vi "FTW-File-TextWrite.vi"(0 "Filepath":path, 5 "Text to Write":string, 7 "Mode":enum16{"Overwrite", "Append"}(ring), 11 "error in":errorcluster) -> (4 "Filepath out":path, 15 "error out":errorcluster)   [LabVIEW 2015]
panel:
  # "Inputs"
  # "Outputs"
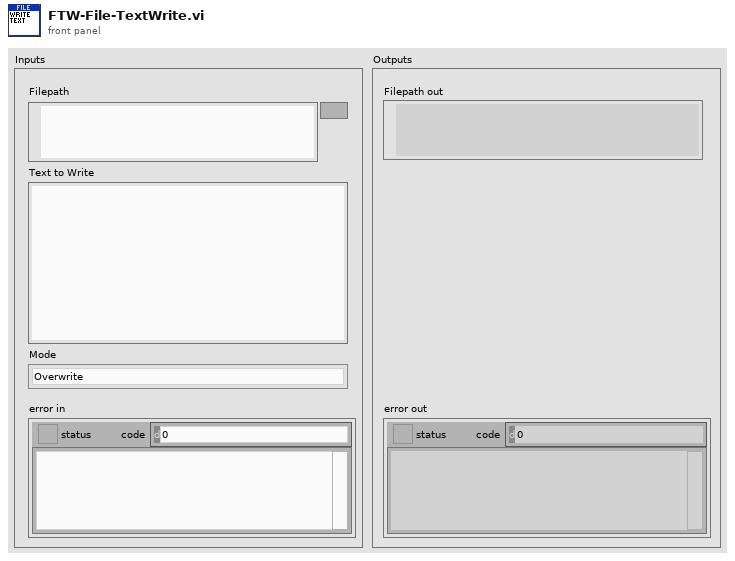
[diagram p1: front panel]
types:
  T1 = enum16{"open", "replace", "create", "open or create", "replace or create", "replace or create with confirmation"}
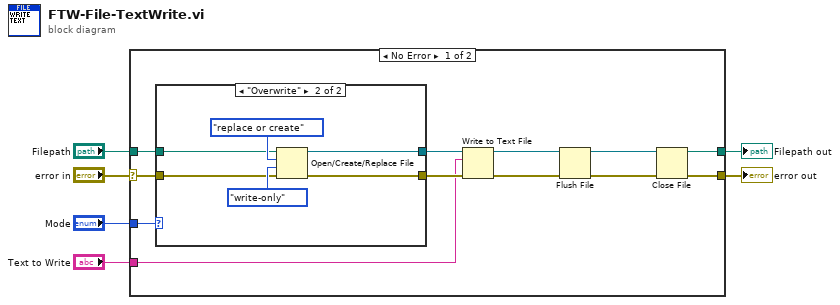
[diagram p0: block diagram]
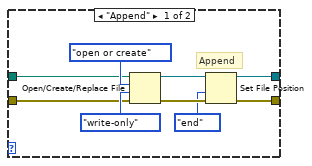
[diagram p2: hidden frame]
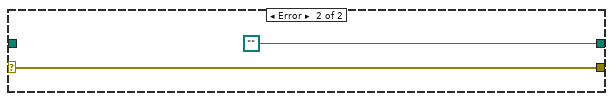
[diagram p3: hidden frame]
diagram:
  n1 = case shown="No Error" "error in" {
    selector: "error in" -> [w10 w34]
    tunnel: "Text to Write" -> [w15 _]
    tunnel: "Filepath" -> [w14 _]
    tunnel: [w13 path ""] -> w4
    tunnel: [w12 w34] -> w3
    tunnel: "Mode" -> [w11 _]
    frame No Error {
      n2 = case shown="\"Overwrite\"" w11 {
        tunnel: [w23 w28] -> w17
        tunnel: [w22 w29] -> w16
        tunnel: w14 -> [w20 w31]
        tunnel: w10 -> [w19 w30]
        frame "Append" {
          # "Append"
          n3 = Open/Create/Replace File(file path (use dialog)=w20, error in=w19, operation (0:open)=T1."open or create", access (0:read/write)=enum16{"read/write", "read-only", "write-only"}."write-only") -> (refnum out=w25:refnum<file>, error out=w24:errorcluster)  [unwired: 2 in, 1 out]
          n4 = Set File Position(refnum=w25, from (0:start)=enum16{"start", "end", "current"}."end", error in=w24) -> (refnum out=w22:refnum<file>, error out=w23:errorcluster)  [unwired: 1 in]
        }
        frame "Overwrite" {
          n5 = Open/Create/Replace File(file path (use dialog)=w31, error in=w30, operation (0:open)=T1."replace or create", access (0:read/write)=enum16{"read/write", "read-only", "write-only"}."write-only") -> (refnum out=w29:refnum<file>, error out=w28:errorcluster)  [unwired: 2 in, 1 out]
        }
      }
      n6 = Write to Text File(file (use dialog)=w16, text=w15, error in=w17) -> (refnum out=w8:refnum<file>, error out=w18:errorcluster)  [unwired: 1 in, 1 out]
      n7 = Flush File(refnum=w8, error in=w18) -> (refnum out=w7:refnum<file>, error out=w9:errorcluster)
      n8 = Close File(refnum=w7, error in=w9) -> (path=w13:path, error out=w12:errorcluster)
    }
    frame Error {
    }
  }
  "error out" <- w3
  "Filepath out" <- w4
